vi "Close.vi"(8 "ErrorIn":errorcluster caption="Error In(no Error)", 11 "ReferenceIn":refnum<class "ErrorDefinitionSQLite.lvclass"> caption="Reference In") -> (0 "ErrorOut":errorcluster caption="Error Out", 3 "ReferenceOut":refnum<class "ErrorDefinitionSQLite.lvclass"> caption="Reference Out")   [LabVIEW 2021, in "ErrorDefinitionSQLite.lvclass"]
uses:
  ErrorDefinitionSQLite.lvclass
  <vilib>/drjdpowell/SQLite Library/SQL Connection/Connection.lvclass
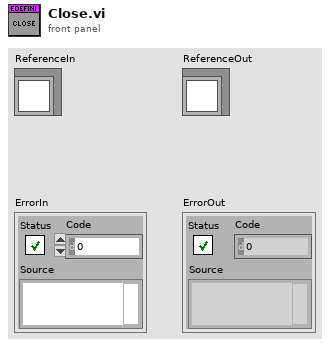
[diagram p1: front panel]
types:
  T1 = typedef "ErrorDefinitionSQLite.lvclass/ObjectAttributes.ctl" = cluster{"Path":path, "SQLiteRef":refnum<class "Connection.lvclass">, "EndOfRange":i32, "DefaultLibrarySize":i32, "StartOfRange":i32}
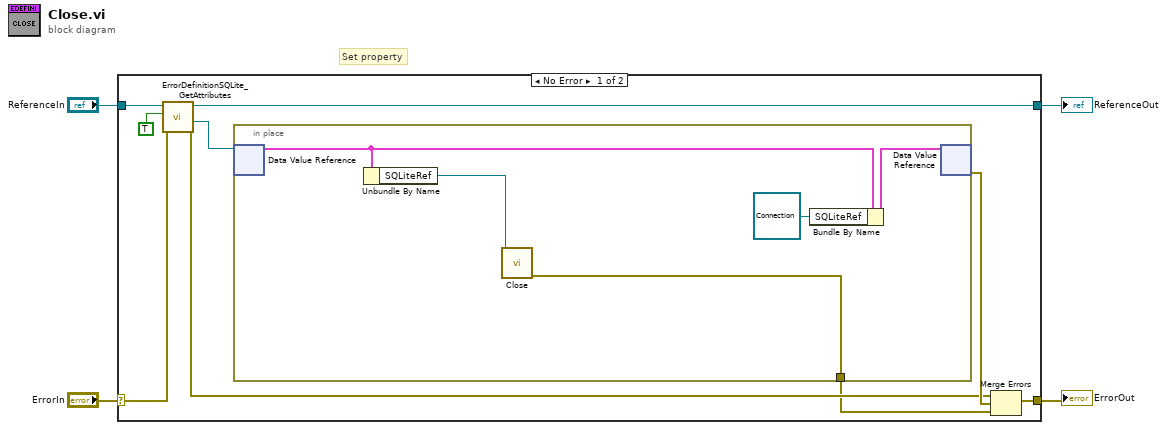
[diagram p0: block diagram]
diagram:
  # "Set property"
  n1 = case shown="No Error" "ErrorIn" {
    selector: "ErrorIn" -> [w8 w20]
    tunnel: [w12 w20] -> w3
    tunnel: [w10 w19] -> w1
    tunnel: "ReferenceIn" -> [w11 w19]
    frame No Error {
      n2 = call "ErrorDefinitionSQLite_GetAttributes.vi"("ErrorIn"=w8, "OnlyGetDVRReference"=TRUE ("OnlyGetDvrReference(False)"), "Reference in"=w11) -> ("ErrorOut"=w7:errorcluster, "DataRef"=w9:refnum<data-value>, "Reference out"=w10:refnum<class "ErrorDefinitionSQLite.lvclass">)  [unwired: 5 in, 1 out]
      n3 = in-place {
        in-place-border: [w16] -> w5
        n4 = in-place-dvr #1(w9) -> (w17:T1)  [unwired: 1 out]
        n5 = Unbundle By Name(w17) -> ("SQLiteRef"=w15:refnum<class "Connection.lvclass">)
        n6 = call-dynamic "Close.vi"("SQLite Connection in"=w15) -> ("error out"=w16:errorcluster)  [unwired: 10 in]
        n7 = Bundle By Name(cluster=w17, "SQLiteRef"=refnum<class "Connection.lvclass"> refnum) -> (w18:T1)
        n8 = in-place-dvr #1(w18) -> (w13:errorcluster)  [unwired: 1 out]
      }
      n9 = Merge Errors(w7, w13, w5) -> (w12:errorcluster)
    }
    frame Error {
    }
  }
  "ErrorOut" <- w3
  "ReferenceOut" <- w1
